vi "Write position Remote.vi"(8 "error in (no error)":errorcluster, 11 "GameEl in":refnum<class "GameEl.lvclass">) -> (0 "error out":errorcluster)   [LabVIEW 2021, in "GameEl.lvclass"]
uses:
  GameEl.lvclass
  GameEl.lvclass/GameEl.ctl
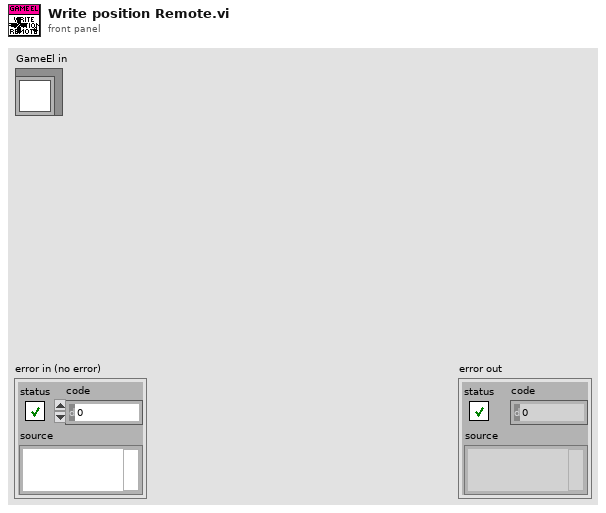
[diagram p1: front panel]
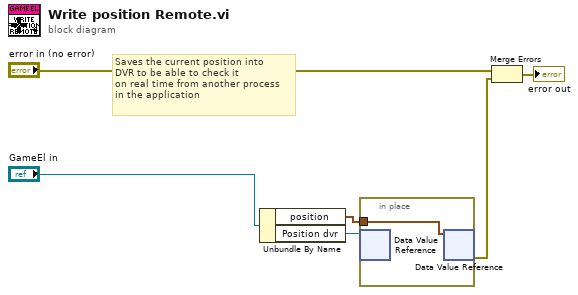
[diagram p0: block diagram]
diagram:
  # "Saves the current position into \nDVR to be able to check it \non real time from another process\nin the application"
  n1 = Unbundle By Name("GameEl in") -> ("position"=w1:cluster{"x":dbl, "y":dbl}[], "Position dvr"=w4:refnum<data-value>)
  n2 = in-place {
    in-place-border: w1 -> [w7]
    n3 = in-place-dvr #1(w4) -> ()  [unwired: 2 out]
    n4 = in-place-dvr #1(w7) -> (w2:errorcluster)  [unwired: 1 out]
  }
  n5 = Merge Errors("error in (no error)", w2) -> (→"error out":errorcluster)
